vi "Render Clear.vi"(8 "error in":errorcluster, 11 "Renderer Pointer":u32 format="%.0x") -> (0 "error out":errorcluster, 3 "return":i32)   [LabVIEW 2015, in "LibSDL2.lvlib"]
uses:
  LibSDL2.lvlib
  DLL/SDL2.dll
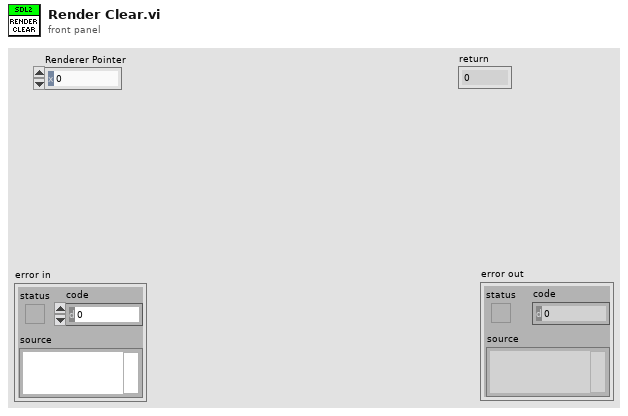
[diagram p1: front panel]
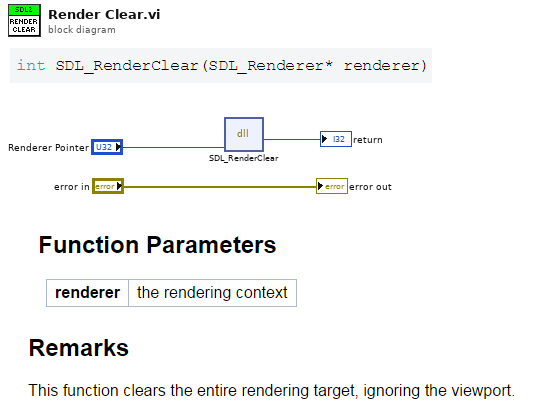
[diagram p0: block diagram]
diagram:
  n1 = dll-call lib="C:/dev/PGS/LabSDL2/Source/Libraries/LibSDL2 Wrapper/DLL/SDL2.dll" fn="SDL_RenderClear"("renderer"="Renderer Pointer") -> ("return type"=→"return":i32)  [unwired: 4 in, 2 out]
  "error out" <- "error in"
